vi "Instrument Message History.vi"(11 "Instrument Message":string) -> (2 "Message Count":i32, 3 "Message History out":string)   [LabVIEW 2026, in "MicroPulse_Driver.lvlib"]
uses:
  MicroPulse_Driver.lvlib
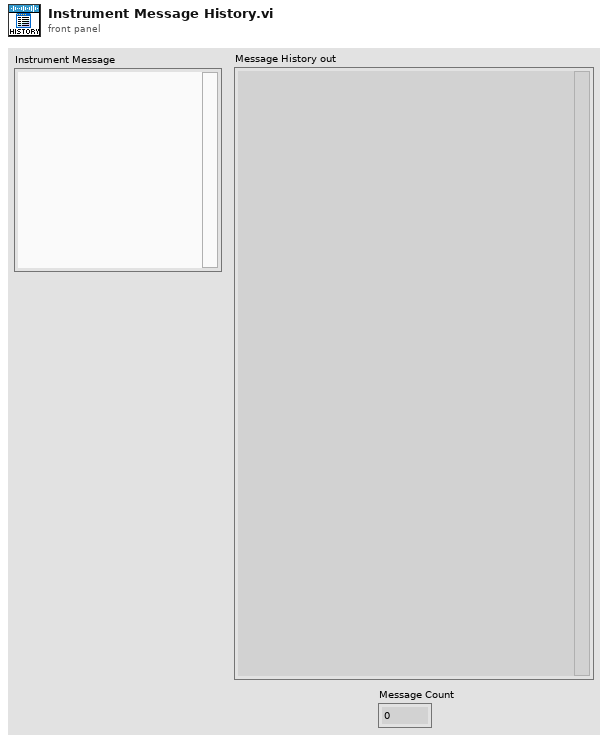
[diagram p1: front panel]
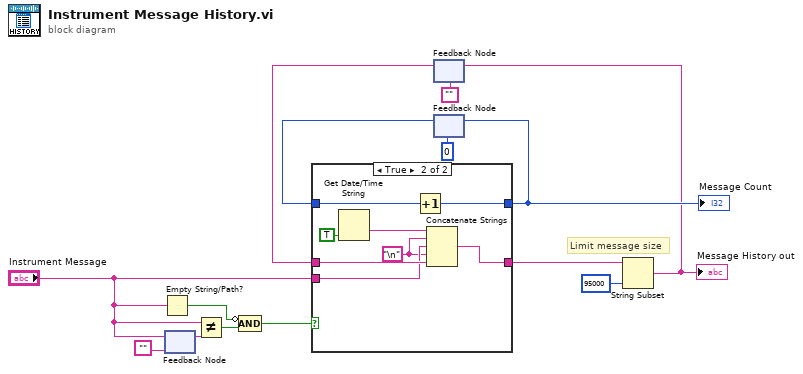
[diagram p0: block diagram]
diagram:
  # "Limit message size"
  n1 = Empty String/Path?(string/path="Instrument Message") -> (empty?=w9:bool)
  n2 = feedback #1("") -> (w12:string)
  n3 = feedback-in #1("Instrument Message") -> ()
  n4 = Not Equal?(x="Instrument Message", y=w12) -> (x != y?=w11:bool)
  n5 = Compound Arithmetic op=AND(invert w9, w11) -> (w10:bool)
  n6 = feedback #2("") -> (w4:string)
  n7 = feedback #3(0) -> (w7:i32)
  n8 = case shown="True" w10 {
    tunnel: "Instrument Message" -> [_ w20]
    tunnel: w4 -> [w16 w21]
    tunnel: [w16 w24] -> w2
    tunnel: [w15 w23] -> w6
    tunnel: w7 -> [w15 w22]
    frame False {
    }
    frame True {
      w19 = "\n"
      n9 = Get Date/Time String(want seconds? (F)=TRUE) -> (time string=w18:string)  [unwired: 2 in, 1 out]
      n10 = Increment(x=w22) -> (x+1=w23:i32)
      n11 = Concatenate Strings(w18, w19, w20, w19, w21) -> (w24:string)
    }
  }
  "Message Count" <- w6
  n12 = feedback-in #3(w6) -> ()
  n13 = String Subset(string=w2, length (rest)=95000 ("y")) -> (substring=w3:string)  [unwired: 1 in]
  "Message History out" <- w3
  n14 = feedback-in #2(w3) -> ()
